vi "State Queue PEEK.vi"(8 "error in (no error)":errorcluster, 11 "State que in":T1[](array[typedef])) -> (0 "error out":errorcluster, 1 "Parameters":variant, 3 "State que out":T1[](array[typedef]), 4 "Empty":bool, 5 "State case out":string)   [LabVIEW 2013, in "State Machine Lib.lvlib"]
doc: "Peeks at the next state on the inputed state queue. Returns if the stack is empty, the state parameter and the original stack."
uses:
  State Machine Lib.lvlib
  STATE cluster.ctl
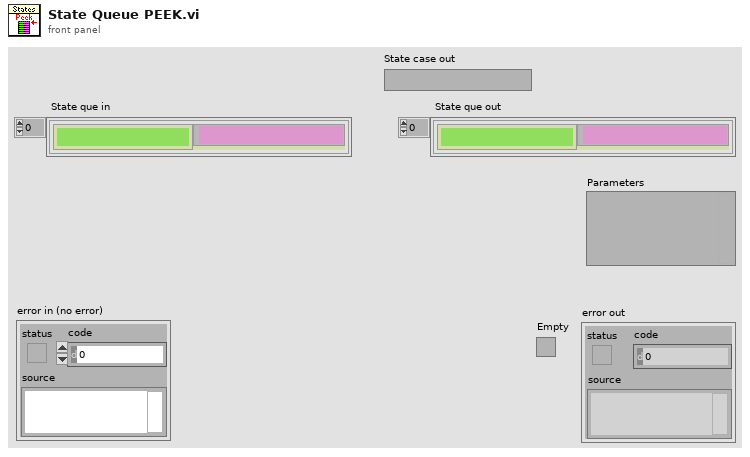
[diagram p1: front panel]
types:
  T1 = typedef "State Machine Lib.lvlib/STATE cluster.ctl" = cluster{"State":string, "Parameters":variant}
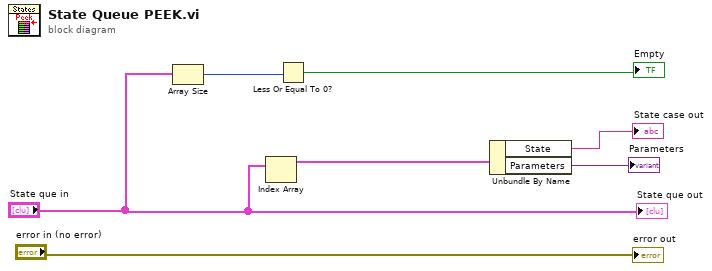
[diagram p0: block diagram]
diagram:
  n1 = Array Size(array="State que in") -> (size(s)=w5:i32)
  n2 = Index Array(array="State que in") -> (element=w3:T1)  [unwired: 1 in]
  n3 = Less Or Equal To 0?(x=w5) -> (x <= 0?=→"Empty":bool)
  n4 = Unbundle By Name(w3) -> ("State"=→"State case out":string, "Parameters"=→"Parameters":variant)
  "error out" <- "error in (no error)"
  "State que out" <- "State que in"
